vi "калькулятор.vi"() -> ()   [LabVIEW 2019]
panel:
  in  "stop":bool
  out "divide":bool
  out "multiply":bool
  out "minus":bool
  out "plus":bool
  in  "divide":bool
  in  "multiply":bool
  in  "minus":bool
  in  "plus":bool
  out "result":dbl
  in  "B":dbl
  in  "A":dbl
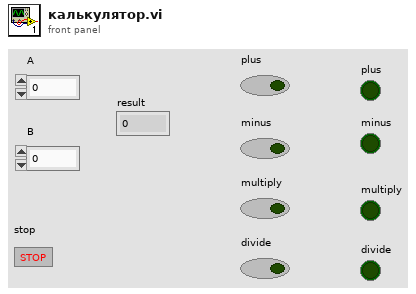
[diagram p1: front panel]
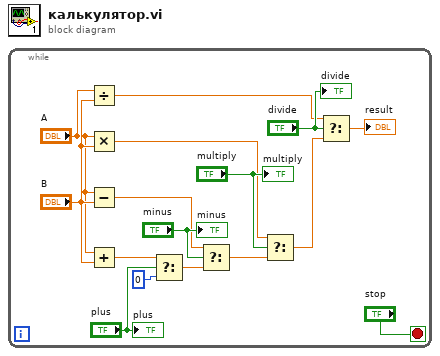
[diagram p0: block diagram]
diagram:
  n1 = while {
    stop <- "stop" stop-if-true
    n2 = Divide(x="A", y="B") -> (x/y=w7:dbl)
    n3 = Multiply(x="A", y="B") -> (x*y=w8:dbl)
    n4 = Subtract(x="A", y="B") -> (x-y=w9:dbl)
    n5 = Add(x="A", y="B") -> (x+y=w10:dbl)
    n6 = Select(t=w10, s="plus", f=0) -> (s? t:f=w6:dbl)
    n7 = Select(t=w9, s="minus", f=w6) -> (s? t:f=w5:dbl)
    n8 = Select(t=w8, s="multiply", f=w5) -> (s? t:f=w4:dbl)
    n9 = Select(t=w7, s="divide", f=w4) -> (s? t:f=→"result":dbl)
    "plus" <- "plus"
    "minus" <- "minus"
    "multiply" <- "multiply"
    "divide" <- "divide"
  }
